vi "SS List Sequencer Configure.vi"(0 "instrument handle":refnum<k15>, 1 "RadioBand (I Agxs An 5ss List Sequencer Setup Radio Band None)":i32(ring) items=["I Agxs An 5ss List Sequencer Setup Radio Band None"=0, "I Agxs An 5ss List Sequencer Setup Radio Bandpgsm"=1, "I Agxs An 5ss List Sequencer Setup Radio Bandegsm"=2, "I Agxs An 5ss List Sequencer Setup Radio Bandrgsm"=3, "I Agxs An 5ss List Sequencer Setup Radio Banddcs1800"=4, "I Agxs An 5ss List Sequencer Setup Radio Bandpcs1900"=5, "I Agxs An 5ss List Sequencer Setup Radio Bandtgsm810"=6, "I Agxs An 5ss List Sequencer Setup Radio Bandgsm450"=7, "I Agxs An 5ss List Sequencer Setup Radio Bandgsm480"=8, "I Agxs An 5ss List Sequencer Setup Radio Bandgsm700"=9, "I Agxs An 5ss List Sequencer Setup Radio Bandgsm850"=10, "I Agxs An 5ss List Sequencer Setup Radio Bandbandi"=11, "I Agxs An 5ss List Sequencer Setup Radio Bandbandii"=12, "I Agxs An 5ss List Sequencer Setup Radio Bandbandiii"=13, "I Agxs An 5ss List Sequencer Setup Radio Bandbandiv"=14, "I Agxs An 5ss List Sequencer Setup Radio Bandbandv"=15, "I Agxs An 5ss List Sequencer Setup Radio Bandbandvi"=16, "I Agxs An 5ss List Sequencer Setup Radio Bandbandvii"=17, "I Agxs An 5ss List Sequencer Setup Radio Bandbandviii"=18, "I Agxs An 5ss List Sequencer Setup Radio Bandbandix"=19, "I Agxs An 5ss List Sequencer Setup Radio Bandbandx"=20, "I Agxs An 5ss List Sequencer Setup Radio Bandbandxi"=21, "I Agxs An 5ss List Sequencer Setup Radio Bandbandxii"=22, "I Agxs An 5ss List Sequencer Setup Radio Bandbandxiii"=23, "I Agxs An 5ss List Sequencer Setup Radio Bandbandxiv"=24, "I Agxs An 5ss List Sequencer Setup Radio Bandbandxix"=25, "I Agxs An 5ss List Sequencer Setup Radio Banduscell"=26, "I Agxs An 5ss List Sequencer Setup Radio Banduspcs"=27, "I Agxs An 5ss List Sequencer Setup Radio Bandjapan"=28, "I Agxs An 5ss List Sequencer Setup Radio Bandkorean"=29, "I Agxs An 5ss List Sequencer Setup Radio Bandnmt"=30, "I Agxs An 5ss List Sequencer Setup Radio Bandimt 2k"=31, "I Agxs An 5ss List Sequencer Setup Radio Bandupper"=32, "I Agxs An 5ss List Sequencer Setup Radio Bandsecond"=33, "I Agxs An 5ss List Sequencer Setup Radio Bandpamr400"=34, "I Agxs An 5ss List Sequencer Setup Radio Bandpamr800"=35, "I Agxs An 5ss List Sequencer Setup Radio Bandimtext"=36, "I Agxs An 5ss List Sequencer Setup Radio Bandpcs 1dot 9g"=37, "I Agxs An 5ss List Sequencer Setup Radio Bandaws"=38, "I Agxs An 5ss List Sequencer Setup Radio Bandus 2dot 5g"=39, "I Agxs An 5ss List Sequencer Setup Radio Bandpublic"=40, "I Agxs An 5ss List Sequencer Setup Radio Bandlower"=41, "I Agxs An 5ss List Sequencer Setup Radio Bandband1"=42, "I Agxs An 5ss List Sequencer Setup Radio Bandband2"=43, "I Agxs An 5ss List Sequencer Setup Radio Bandband3"=44, "I Agxs An 5ss List Sequencer Setup Radio Bandband4"=45, "I Agxs An 5ss List Sequencer Setup Radio Bandband5"=46, "I Agxs An 5ss List Sequencer Setup Radio Bandband6"=47, "I Agxs An 5ss List Sequencer Setup Radio Bandband7"=48, "I Agxs An 5ss List Sequencer Setup Radio Bandband8"=49, "I Agxs An 5ss List Sequencer Setup Radio Bandbanda"=87, "I Agxs An 5ss List Sequencer Setup Radio Bandband10"=50, "I Agxs An 5ss List Sequencer Setup Radio Bandband11"=51, "I Agxs An 5ss List Sequencer Setup Radio Bandband12"=52, "I Agxs An 5ss List Sequencer Setup Radio Bandband13"=53, "I Agxs An 5ss List Sequencer Setup Radio Bandband14"=54, "I Agxs An 5ss List Sequencer Setup Radio Bandbandb"=88, "I Agxs An 5ss List Sequencer Setup Radio Bandbandc"=89, "I Agxs An 5ss List Sequencer Setup Radio Bandband17"=55, "I Agxs An 5ss List Sequencer Setup Radio Bandband18"=56, "I Agxs An 5ss List Sequencer Setup Radio Bandband19"=57, "I Agxs An 5ss List Sequencer Setup Radio Bandband20"=58, "I Agxs An 5ss List Sequencer Setup Radio Bandband21"=59, "I Agxs An 5ss List Sequencer Setup Radio Bandbandd"=90, "I Agxs An 5ss List Sequencer Setup Radio Bandbande"=91, "I Agxs An 5ss List Sequencer Setup Radio Bandband24"=60, "I Agxs An 5ss List Sequencer Setup Radio Bandband25"=61, "I Agxs An 5ss List Sequencer Setup Radio Bandband26"=62, "I Agxs An 5ss List Sequencer Setup Radio Bandband27"=63, "I Agxs An 5ss List Sequencer Setup Radio Bandband28"=64, "I Agxs An 5ss List Sequencer Setup Radio Bandband29"=65, "I Agxs An 5ss List Sequencer Setup Radio Bandband30"=66, "I Agxs An 5ss List Sequencer Setup Radio Bandband31"=67, "I Agxs An 5ss List Sequencer Setup Radio Bandband65"=68, "I Agxs An 5ss List Sequencer Setup Radio Bandband66"=69, "I Agxs An 5ss List Sequencer Setup Radio Bandband68"=70, "I Agxs An 5ss List Sequencer Setup Radio Bandband252"=71, "I Agxs An 5ss List Sequencer Setup Radio Bandband255"=72, "I Agxs An 5ss List Sequencer Setup Radio Bandband33"=73, "I Agxs An 5ss List Sequencer Setup Radio Bandband34"=74, "I Agxs An 5ss List Sequencer Setup Radio Bandband35"=75, "I Agxs An 5ss List Sequencer Setup Radio Bandband36"=76, "I Agxs An 5ss List Sequencer Setup Radio Bandband37"=77, "I Agxs An 5ss List Sequencer Setup Radio Bandband38"=78, "I Agxs An 5ss List Sequencer Setup Radio Bandband39"=79, "I Agxs An 5ss List Sequencer Setup Radio Bandband40"=80, "I Agxs An 5ss List Sequencer Setup Radio Bandband41"=81, "I Agxs An 5ss List Sequencer Setup Radio Bandband42"=82, "I Agxs An 5ss List Sequencer Setup Radio Bandband43"=83, "I Agxs An 5ss List Sequencer Setup Radio Bandband44"=84, "I Agxs An 5ss List Sequencer Setup Radio Bandband45"=85, "I Agxs An 5ss List Sequencer Setup Radio Bandband46"=86, "I Agxs An 5ss List Sequencer Setup Radio Bandbandf"=92], 2 "Frequency":dbl caption="Frequency (Hz)", 3 "Waveform":string, 5 "StepIndex":i32 format="%.0g", 6 "Time":dbl, 7 "TriggerType (I Agxs An 5ss List Sequencer Setup Input Trigger Type Free Run)":i32(ring) items=["I Agxs An 5ss List Sequencer Setup Input Trigger Type Free Run", "I Agxs An 5ss List Sequencer Setup Input Trigger Type Internal", "I Agxs An 5ss List Sequencer Setup Input Trigger Type Manual", "I Agxs An 5ss List Sequencer Setup Input Trigger Type Bus", "I Agxs An 5ss List Sequencer Setup Input Trigger Type External2", "I Agxs An 5ss List Sequencer Setup Input Trigger Type External4"], 8 "OutputTriggerEnabled (Off)":bool, 9 "TransitionTime":dbl caption="TransitionTime (sec)", 10 "Count":i32 format="%.0g", 11 "error in (no error)":errorcluster {"code" format="%.0x"}, 12 "Link (Ss List Sequencer Setup Radio Band Link Uplink)":i32(ring) items=["Ss List Sequencer Setup Radio Band Link Uplink", "Ss List Sequencer Setup Radio Band Link Downlink"], 13 "Amplitude":dbl caption="Amplitude(dBm)", 14 "StepDuration (Ss List Sequencer Step Duration Type Time)":i32(ring) items=["Ss List Sequencer Step Duration Type Time", "Ss List Sequencer Step Duration Type Continuous", "Ss List Sequencer Step Duration Type Count"]) -> (4 "instrument handle out":refnum<k15>, 15 "error out":errorcluster {"code" format="%.0x"})   [LabVIEW 2009, in "Keysight XSAn.lvlib"]
doc: "Configure the List Sequencer.\n\nSupported Models: M8920A, M9420A, M9421A."
uses:
  <instrlib>/Keysight XSAn/Keysight XSAn.lvlib
  AgXSAn.dll
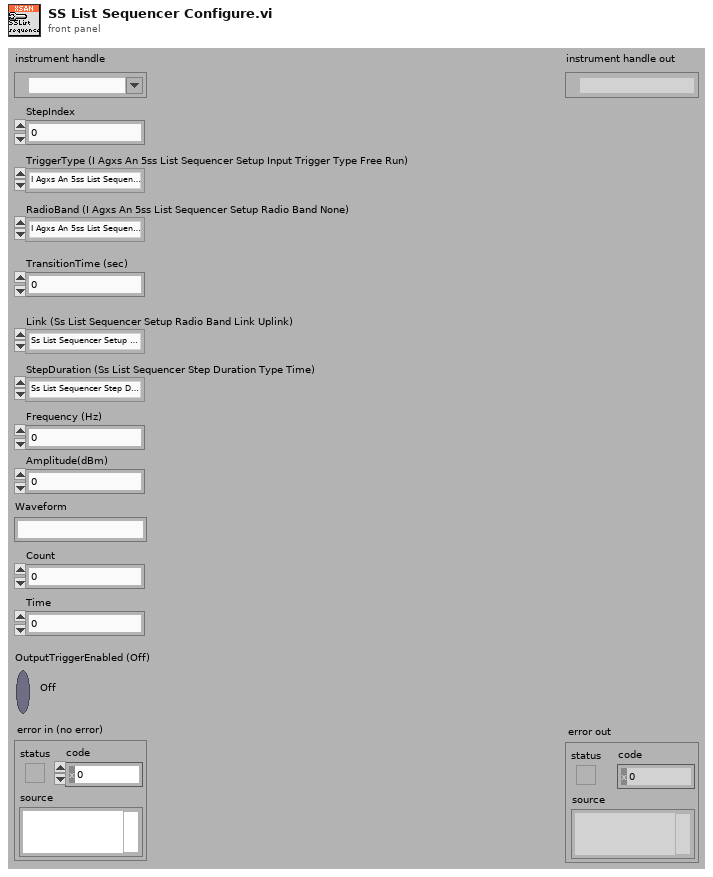
[diagram p1: front panel]
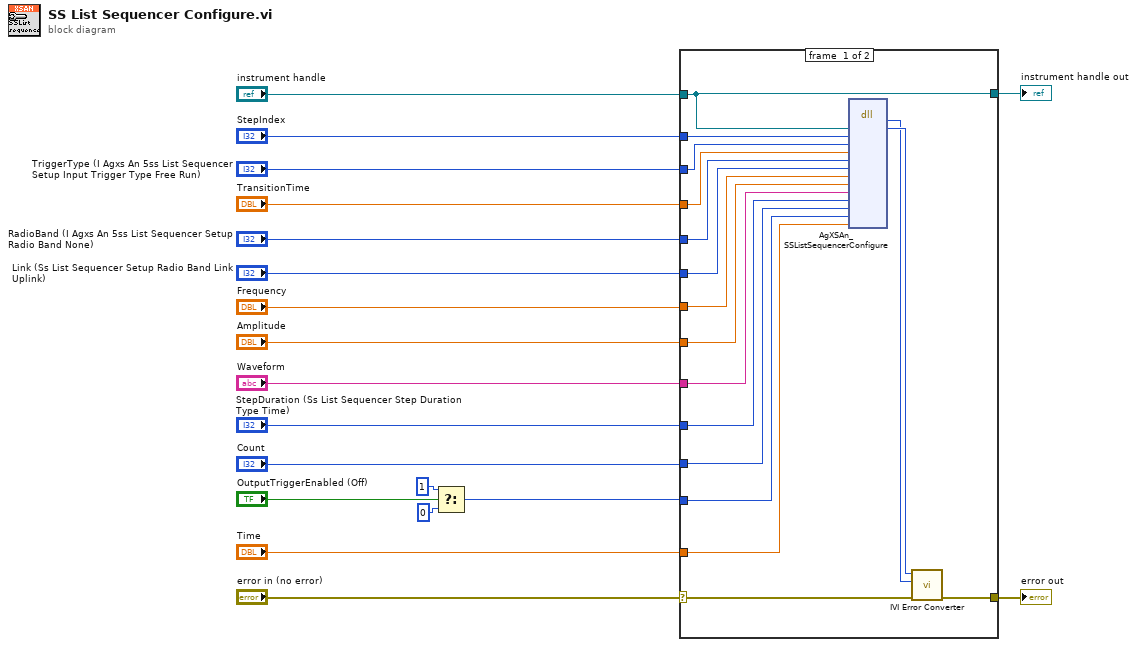
[diagram p0: block diagram]
diagram:
  n1 = Select(t=u16 1, s="OutputTriggerEnabled (Off)", f=u16 0) -> (s? t:f=w3:u16)
  n2 = case shown="No Error" "error in (no error)" {
    selector: "error in (no error)" -> [w34 w38]
    tunnel: [w33 w38] -> w19
    tunnel: "instrument handle" -> [w21 w37]
    tunnel: "StepIndex" -> [w32 _]
    tunnel: "TriggerType (I Agxs An 5ss List Sequencer Setup Input Trigger Type Free Run)" -> [w31 _]
    tunnel: "TransitionTime" -> [w30 _]
    tunnel: "RadioBand (I Agxs An 5ss List Sequencer Setup Radio Band None)" -> [w29 _]
    tunnel: "Link (Ss List Sequencer Setup Radio Band Link Uplink)" -> [w28 _]
    tunnel: "Frequency" -> [w27 _]
    tunnel: "Amplitude" -> [w26 _]
    tunnel: "Waveform" -> [w25 _]
    tunnel: "StepDuration (Ss List Sequencer Step Duration Type Time)" -> [w24 _]
    tunnel: "Count" -> [w20 _]
    tunnel: w3 -> [w23 _]
    tunnel: "Time" -> [w22 _]
    tunnel: [w21 w37] -> w1
    frame #0 {
      n3 = dll-call lib="AgXSAn**.dll" fn="AgXSAn_SSListSequencerConfigure"("Vi"=w21, "StepIndex"=w32, "TriggerType"=w31, "TransitionTime"=w30, "RadioBand"=w29, "Link"=w28, "Frequency"=w27, "Amplitude"=w26, "Waveform"=w25, "StepDuration"=w24, "Count"=w20, "OutputTriggerEnabled"=w23, "Time"=w22) -> (w35:i32, "Vi"=w36:u32)  [unwired: 15 in, 2 out]
      n4 = call <instrlib>:"IVI Error Converter.vi"("error in (no error)"=w34, "IVI error code (0)"=w35, "instrument handle"=w36) -> ("error out"=w33:errorcluster)  [unwired: 7 in, 1 out]
    }
    frame #1 {
    }
  }
  "error out" <- w19
  "instrument handle out" <- w1
